vi "Read Description.vi"(11 "Milk in":refnum<class "Milk.lvclass">) -> (2 "Description":string, 3 "Milk out":refnum<class "Milk.lvclass">)   [LabVIEW 2020, in "Milk.lvclass"]
uses:
  Milk.lvclass
  Milk.lvclass/Milk.ctl
  Beverage.lvclass
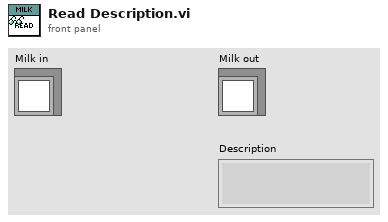
[diagram p1: front panel]
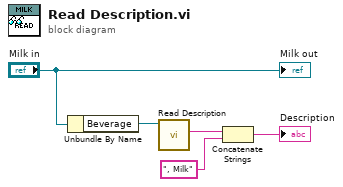
[diagram p0: block diagram]
diagram:
  n1 = Unbundle By Name("Milk in") -> ("Beverage"=w4:refnum<class "Beverage.lvclass">)
  n2 = call-dynamic "Read Description.vi"("Beverage in"=w4) -> ("Description"=w3:string)  [unwired: 9 in, 1 out]
  n3 = Concatenate Strings(w3, ", Milk" ("string")) -> (→"Description":string)
  "Milk out" <- "Milk in"
